vi "get_phase_shift.vi"(8 "error in (no error)":errorcluster, 11 "TrajectoryDL110420DoubleCircle in":refnum<class "TrajectoryDL110420DoubleCircle.lvclass">) -> (0 "error out":errorcluster, 2 "phase shift":dbl, 3 "TrajectoryDL110420DoubleCircle out":refnum<class "TrajectoryDL110420DoubleCircle.lvclass">)   [LabVIEW 2010, in "TrajectoryDL110420DoubleCircle.lvclass"]
uses:
  TrajectoryDL110420DoubleCircle.lvclass
  common/classes/SpaceVector/SpaceVector/SpaceVector.lvclass
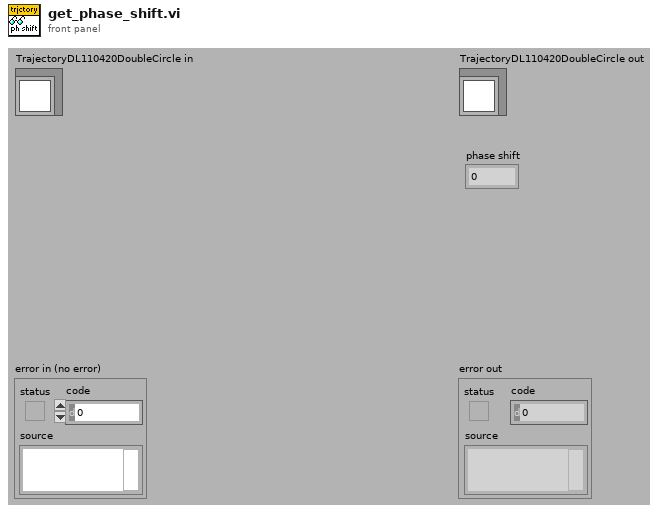
[diagram p1: front panel]
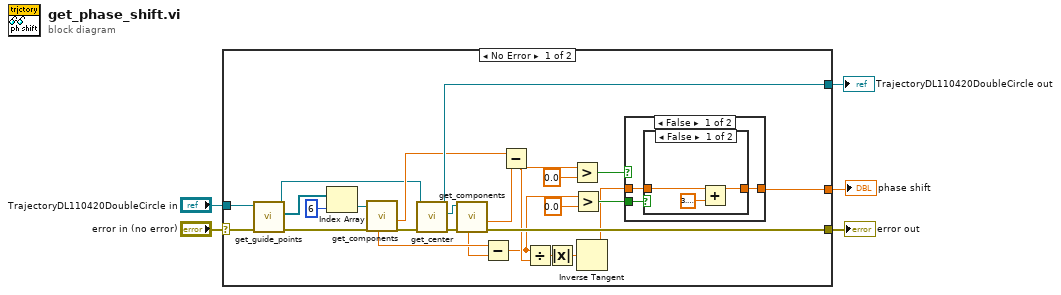
[diagram p0: block diagram]
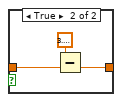
[diagram p2: hidden frame]
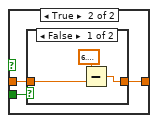
[diagram p3: hidden frame]
diagram:
  n1 = case shown="No Error" "error in (no error)" {
    selector: "error in (no error)" -> [w7 w49]
    tunnel: [w27 w49] -> w4
    tunnel: [w26 w48] -> w2
    tunnel: "TrajectoryDL110420DoubleCircle in" -> [w9 w48]
    tunnel: [w11 _] -> w1
    frame No Error {
      n2 = call-dynamic "get_guide_points.vi"("error in (no error)"=w7, "TrajectoryDL110420DoubleCircle in"=w9) -> ("error out"=w6:errorcluster, "guide points"=w10:refnum<class "SpaceVector.lvclass">[], "TrajectoryDL110420DoubleCircle out"=w8:refnum<class "TrajectoryDL110420DoubleCircle.lvclass">)  [unwired: 7 in]
      n3 = Index Array(array=w10, index=6) -> (element=w30:refnum<class "SpaceVector.lvclass">)
      n4 = call "get_components.vi"("error in (no error)"=w6, "SpaceVector in"=w30) -> ("error out"=w28:errorcluster, "x"=w21:dbl[unit], "y"=w24:dbl[unit])  [unwired: 4 in, 3 out]
      n5 = call-dynamic "get_center.vi"("error in (no error)"=w28, "TrajectoryDL110420DoubleCircle in"=w8) -> ("error out"=w29:errorcluster, "center"=w25:refnum<class "SpaceVector.lvclass">, "TrajectoryDL110420DoubleCircle out"=w26:refnum<class "TrajectoryDL110420DoubleCircle.lvclass">)  [unwired: 7 in]
      n6 = call "get_components.vi"("error in (no error)"=w29, "SpaceVector in"=w25) -> ("error out"=w27:errorcluster, "x"=w22:dbl[unit], "y"=w23:dbl[unit])  [unwired: 4 in, 3 out]
      n7 = Subtract(x=w24, y=w23) -> (x-y=w15:dbl[unit])
      n8 = Subtract(x=w21, y=w22) -> (x-y=w18:dbl[unit])
      n9 = Divide(x=w15, y=w18) -> (x/y=w20:dbl)
      n10 = Absolute Value(x=w20) -> (abs(x)=w19:dbl)
      n11 = Greater?(x=w18, y=dbl[unit] 0.0) -> (0:w14:bool)
      n12 = Greater?(x=w15, y=dbl[unit] 0.0) -> (0:w13:bool)
      n13 = Inverse Tangent(1:w19) -> (0:w12:dbl)
      n14 = case shown="False" w14 {
        tunnel: w13 -> [w34 w43]
        tunnel: w12 -> [w33 w42]
        tunnel: [w32 w41] -> w11
        frame False {
          n15 = case shown="False" w34 {
            tunnel: w33 -> [w37 w39]
            tunnel: [w35 w38] -> w32
            frame False {
              n16 = Add(x=w37, y=3.141592653589793) -> (x+y=w35:dbl)
            }
            frame True {
              n17 = Subtract(x=3.141592653589793, y=w39) -> (x-y=w38:dbl)
            }
          }
        }
        frame True {
          n18 = case shown="False" w43 {
            tunnel: w42 -> [w45 w47]
            tunnel: [w44 w47] -> w41
            frame False {
              n19 = Subtract(x=6.283185307179586, y=w45) -> (x-y=w44:dbl)
            }
            frame True {
            }
          }
        }
      }
    }
    frame Error {
    }
  }
  "error out" <- w4
  "TrajectoryDL110420DoubleCircle out" <- w2
  "phase shift" <- w1
